vi "test VIT Verify Person.vi"(8 "error in":errorcluster, 11 "Testing Approval Tests in":refnum<class "VITester Extension Tests.lvclass">) -> (0 "error out":errorcluster, 3 "Testing Approval Tests out":refnum<class "VITester Extension Tests.lvclass">)   [LabVIEW 2026, in "VITester Extension Tests.lvclass"]
uses:
  VITester Extension Tests.lvclass
  Common/Person/Person.lvclass
  Common/Person/Person.lvclass/Person.ctl
  Source/Approval Tests/Options/Options.lvclass/Options.ctl
  Source/Approval Tests/Naming Data/Naming Data.lvclass/Naming Data.ctl
  d04af62d-be56-4854-8c3c-5601869294bc.vi
  Common/Person/Write First Name.vi
  Common/Person/Write Last Name.vi
  Common/Person/Write Title.vi
  d04af62d-be56-4854-8c3c-5601869294bc.vi/ef028380-787c-4fa5-86c8-b0b7860ce2dc.vi
  Source/Approval Tests/Replace if Empty.vi
  Source/Approval Tests/Update Test Name if Not Defined.vi
  Source/Approval Tests/Verify Core.vi
  d04af62d-be56-4854-8c3c-5601869294bc.vi/ef028380-787c-4fa5-86c8-b0b7860ce2dc.vi/93c5622b-9fb7-41e0-8c76-3fde37e94e34.vi
  Source/Approval Tests/Options/Read Scrubber.vi
  Source/Approval Tests/Naming Data/Read Test VI Name.vi
  Source/Approval Tests/Naming Data/Write Test VI Name.vi
  Source/Approval Tests/Options/Read Namer.vi
  Source/Approval Tests/Options/Read Naming Data.vi
  Source/Approval Tests/Options/Read Reporter.vi
  Source/Approval Tests/Options/Read Text Comparator.vi
  d04af62d-be56-4854-8c3c-5601869294bc.vi/ef028380-787c-4fa5-86c8-b0b7860ce2dc.vi/93c5622b-9fb7-41e0-8c76-3fde37e94e34.vi/04cb982b-2eda-40d0-8d7e-90f8e0b569b2.vi
  d04af62d-be56-4854-8c3c-5601869294bc.vi/ef028380-787c-4fa5-86c8-b0b7860ce2dc.vi/93c5622b-9fb7-41e0-8c76-3fde37e94e34.vi/04cb982b-2eda-40d0-8d7e-90f8e0b569b2.vi/04ec6d97-7b7c-4123-b264-4b7eb8a41208.vi
  <vilib>/PNR/JSONtext Object Serialization/Generic Object Serializer/Generic Object Serializer.lvclass
  Source/Approval Tests/Options/Add Label to Namer.vi
  <vilib>/JDP Science/JSONtext/Variant to JSON Text.vi
  Source/Approval Tests/conv EOL.vi
  <vilib>/Utility/libraryn.llb/Check if File or Folder Exists.vi
  Source/Approval Tests/Reporter/Report.vi
  Source/Approval Tests/Options/Options.lvclass
  Source/Approval Tests/Scrubber/Scrubber.lvclass
  Source/Approval Tests/Namer/Namer.lvclass
  Source/Approval Tests/Naming Data/Naming Data.lvclass
  Source/Approval Tests/Reporter/Reporter.lvclass
  Source/Approval Tests/Text Comparator/Text Comparator.lvclass
  VITester Extension Tests.lvclass/VITester Extension Tests.ctl
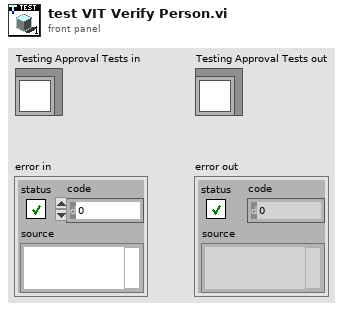
[diagram p1: front panel]
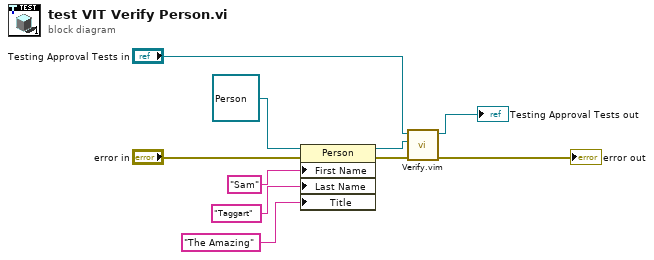
[diagram p0: block diagram]
diagram:
  n1 = property class="Person"(reference=refnum<class "Person.lvclass"> refnum ("Person.lvclass"), error in="error in", "First Name"="Sam", "Last Name"="Taggart", "Title"="The Amazing") -> (reference out=w1:refnum<class "Person.lvclass">, error out=w8:errorcluster)
  n2 = call "Verify.vim"("error in"=w8, "Test Data"=w1, "TestCase in"="Testing Approval Tests in") -> ("error out"=→"error out":errorcluster, "TestCase out"=→"Testing Approval Tests out":refnum<class "VITester Extension Tests.lvclass">)  [unwired: 7 in]
